vi "Read Position.vi"(8 "error in (no error)":errorcluster, 11 "Fruit in":refnum<class "Fruit.lvclass">) -> (0 "error out":errorcluster, 2 "Position":cluster{"X":dbl, "Y":dbl}, 3 "Fruit out":refnum<class "Fruit.lvclass">)   [LabVIEW 2021]
uses:
  Fruit.lvclass
  C:/Users/poche/Programs/LabVIEW/Snake Game/GameEl_class/GameEl.lvclass
  C:/Users/poche/Programs/LabVIEW/Snake Game/Fruit_class/Fruit.lvclass
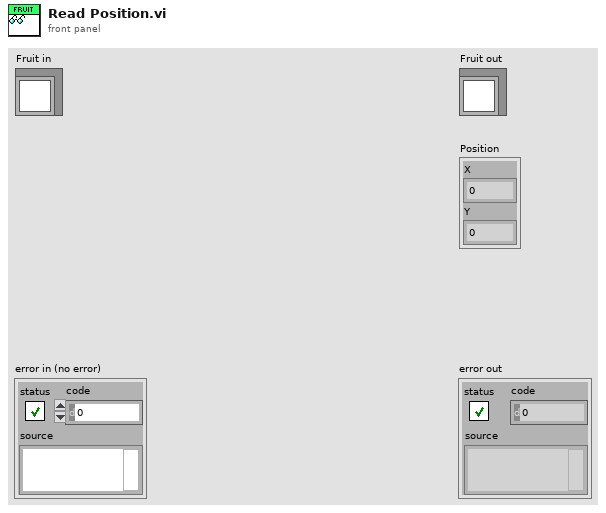
[diagram p1: front panel]
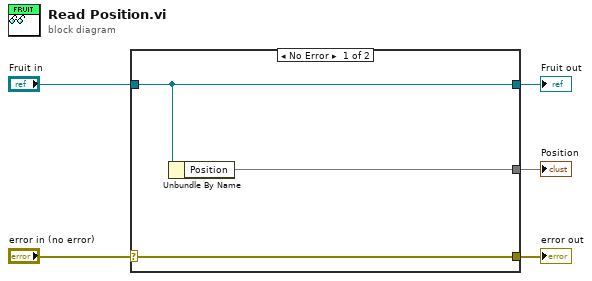
[diagram p0: block diagram]
diagram:
  n1 = case shown="No Error" "error in (no error)" {
    selector: "error in (no error)" -> [w8 w9]
    tunnel: [w8 w9] -> w4
    tunnel: [w7 w10] -> w2
    tunnel: "Fruit in" -> [w7 w10]
    tunnel: [w6 _] -> w1
    frame No Error {
      n2 = Unbundle By Name(w7) -> ("Position"=w6)
    }
    frame Error {
    }
  }
  "error out" <- w4
  "Fruit out" <- w2
  "Position" <- w1
